vi "Test StatusHistory.vi"() -> (0 "error out":errorcluster, 3 "StatusHistory out":refnum<class "StatusHistory.lvclass">)   [LabVIEW 2015, in "StatusHistory.lvclass"]
doc: "<b> </b> <b> </b>\n©2016 Q Software Innovations, LLC (QSI)\nwritten by Quentin Alldredge\nproduced in LabVIEW 2015\n\nsupport@qsoftwareinnovations.com\nwww.qsoftwareinnovations.com\n\nAll rights reserved.\n\nRedistribution and use in source and binary forms, with or without modification, are permitted provided that the following conditions are met:\n\n * Redistributions of source code must retain the above copyright notice, this list of conditions and the following disclaimer.\n * Redistributions in binary form must reproduce the above copyright notice, this list of conditions and the following disclaimer in the documentation and/or other materials provided with the distribution.\n * Neither the name of Q Software Innovations, LLC. nor the names of its contributors may be used to endorse or promote products derived from this software without specific prior written permission.\n\nTHIS SOFTWARE IS PROVIDED BY THE COPYRIGHT HOLDERS AND CONTRIBUTORS \"AS IS\" AND ANY EXPRESS OR IMPLIED WARRANTIES, INCLUDING, BUT NOT LIMITED TO, THE IMPLIED WARRANTIES OF MERCHANTABILITY AND FITNESS FOR A PARTICULAR PURPOSE ARE DISCLAIMED. IN NO EVENT SHALL THE COPYRIGHT OWNER OR CONTRIBUTORS BE LIABLE FOR ANY DIRECT, INDIRECT, INCIDENTAL, SPECIAL, EXEMPLARY, OR CONSEQUENTIAL DAMAGES (INCLUDING, BUT NOT LIMITED TO, PROCUREMENT OF SUBSTITUTE GOODS OR SERVICES; LOSS OF USE, DATA, OR PROFITS; OR BUSINESS INTERRUPTION) HOWEVER CAUSED AND ON ANY THEORY OF LIABILITY, WHETHER IN CONTRACT, STRICT LIABILITY, OR TORT (INCLUDING NEGLIGENCE OR OTHERWISE) ARISING IN ANY WAY OUT OF THE USE OF THIS SOFTWARE, EVEN IF ADVISED OF THE POSSIBILITY OF SUCH DAMAGE."
uses:
  StatusHistory.lvclass
  Direction.ctl
  Write Most Recent Color.vi
  Write Least Recent Color.vi
  Write History Size.vi
  Write Direction.vi
panel:
  in  "Direction":T1
  in  "History Size":u32
  in  "Least Recent Color":u32(colorbox)
  in  "Most Recent Color":u32(colorbox)
  in  "String":string
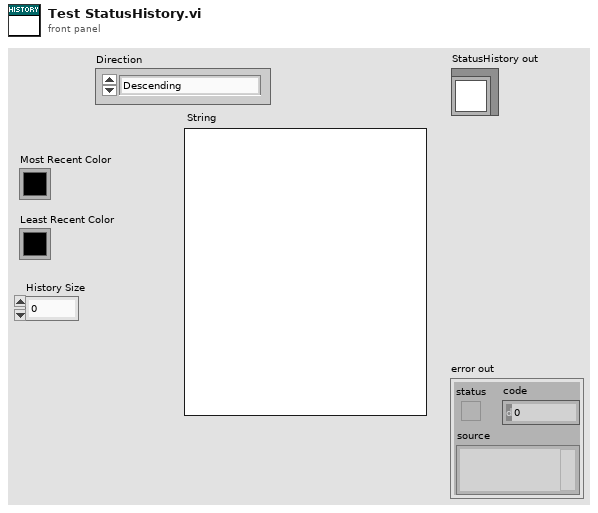
[diagram p1: front panel]
types:
  T1 = typedef "StatusHistory.lvclass/Direction.ctl" = enum16{"Descending", "Ascending"}
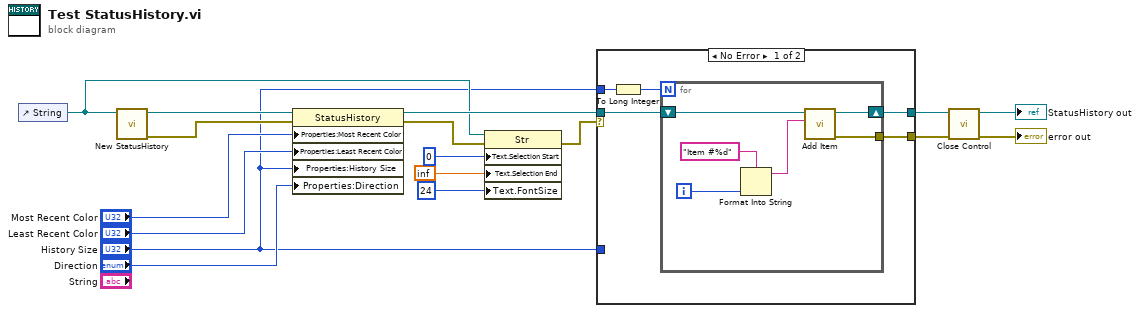
[diagram p0: block diagram]
diagram:
  n1 = control-ref of="String"() -> (w4:refnum<vi>)
  n2 = call "New StatusHistory.vi"("Reference"=w4) -> ("error out"=w2:errorcluster, "StatusHistory out"=w3:refnum<class "StatusHistory.lvclass">)  [unwired: 9 in]
  n3 = property class="StatusHistory"(reference=w3, error in=w2, "Properties:Most Recent Color"="Most Recent Color", "Properties:Least Recent Color"="Least Recent Color", "Properties:History Size"="History Size", "Properties:Direction"="Direction") -> (reference out=w17:refnum<class "StatusHistory.lvclass">, error out=w8:errorcluster)
  n4 = property class="Str"(reference=w4, error in=w8, "Text.Selection Start"=u32 0 ("Text.Selection:Start"), "Text.Selection End"=inf, "Text.FontSize"=u32 24 ("Text.Font:Size")) -> (error out=w7:errorcluster)  [unwired: 1 out]
  n5 = case shown="No Error" w7 {
    selector: w7 -> [_ w30]
    tunnel: [w20 w30] -> w10
    tunnel: [w21 w29] -> w12
    tunnel: w17 -> [w22 w29]
    tunnel: "History Size" -> [_ _]
    tunnel: "History Size" -> [w19 _]
    frame No Error {
      n6 = To Long Integer(number=w19) -> (32bit integer=w18:i32)
      n7 = for {
        N: w18 -> [_]
        shift-right: [w27] -> w21
        shift-left: w22 -> [w28]
        tunnel: [w26] -> w20
        i -> [w24]
        n8 = Format Into String(format string="Item #%d", w24) -> (resulting string=w25:string)  [unwired: 2 in, 1 out]
        n9 = call "Add Item.vi"("Item to Add"=w25, "StatusHistory in"=w28) -> ("error out"=w26:errorcluster, "StatusHistory out"=w27:refnum<class "StatusHistory.lvclass">)  [unwired: 8 in]
      }
    }
    frame Error {
    }
  }
  n10 = call-dynamic "Close Control.vi"("error in (no error)"=w10, "StatusHistory in"=w12) -> ("error out"=→"error out":errorcluster, "StatusHistory out"=→"StatusHistory out":refnum<class "StatusHistory.lvclass">)  [unwired: 8 in]
